vi "Agilent Extract Gain Offset.vi"(8 "Error In":errorcluster, 11 "Gain/Offset":string) -> (0 "Error Out":errorcluster, 3 "Gain/Offset out":dbl)   [LabVIEW 2023]
uses:
  <vilib>/Utility/error.llb/whitespace.ctl
  <vilib>/Utility/error.llb/Trim Whitespace One-Sided.vi
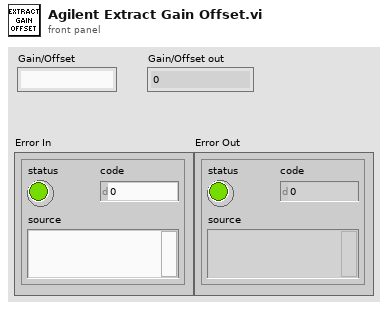
[diagram p1: front panel]
types:
  T1 = typedef "whitespace.ctl" = u16
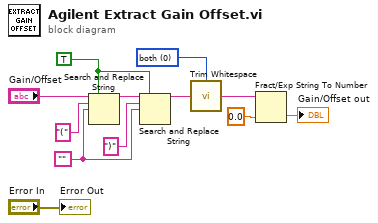
[diagram p0: block diagram]
diagram:
  w4 = T1 0 items=["both", "start of string", "end of string"] ("location (both)")
  w6 = TRUE ("replace all? (F)")
  w8 = ""
  n1 = Search and Replace String(replace all?=w6, input string="Gain/Offset", search string="(", replace string=w8) -> (result string=w9:string)  [unwired: 4 in, 3 out]
  n2 = Search and Replace String(replace all?=w6, input string=w9, search string=")", replace string=w8) -> (result string=w5:string)  [unwired: 4 in, 3 out]
  n3 = call <vilib>:"Trim Whitespace.vi"("string"=w5, "location (both)"=w4) -> ("trimmed string"=w3:string)
  n4 = Fract/Exp String To Number(string=w3, default (0 dbl)=0.0 ("default (0 DBL)")) -> (number=→"Gain/Offset out":dbl)  [unwired: 2 in, 1 out]
  "Error Out" <- "Error In"
